vi "GetNodeList.vi"(8 "Status":T4[](array[typedef]), 10 "servers":T3[](array[typedef])) -> (1 "Topic Types":string[](array[string]), 3 "Published Topics":string[](array[string]))   [LabVIEW 2012]
doc: "Gets all topics that are published by this node."
uses:
  <userlib>/rosforlv/ROS/Code/Console/Servers/ServerSubs/MyState.ctl
  <userlib>/rosforlv/ROS/Code/Console/Servers/ServerSubs/ServoInfo.ctl
  <userlib>/rosforlv/ROS/Code/SubVIs/_ROSControl.ctl
  <userlib>/rosforlv/ROS/Code/SubVIs/_ROSDirection.ctl
panel:
  in  "ROS.Direction":T1
  in  "Node ROS":T2={"topic port"=0, "Node"="", "topic"="", "type"="", "node port"=0, "error "={"status"=FALSE, "code"=0, "source"=""}, "Direction"=enum."Node", "APIs"=[], "Update (ms)"=1, "write queue"=1}
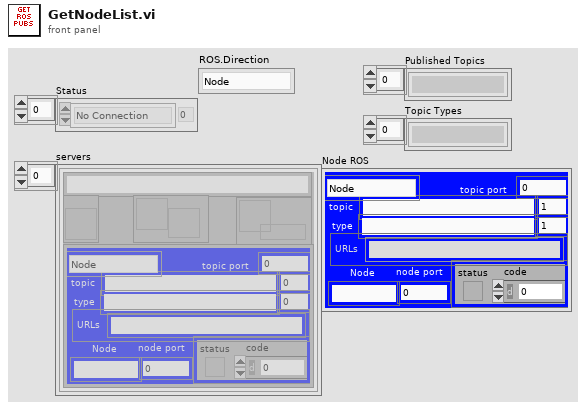
[diagram p1: front panel]
types:
  T1 = typedef "_ROSDirection.ctl" = enum16{"Node", "Publisher", "Subscriber", "Service Client"}
  T2 = typedef "_ROSControl.ctl" = cluster{"topic port":u16, "Node":string, "topic":string, "type":string, "node port":u32, "error ":errorcluster, "Direction":T1, "APIs":string[], "Update (ms)":u16, "write queue":u16}
  T3 = typedef "ServoInfo.ctl" = cluster{"vi name":string, "VI Refnum":refnum<vi>, "queue":refnum<queue>, "ROS":T2, "notifier":refnum<notifier>}
  T4 = typedef "MyState.ctl" = enum16{"No Connection", "Registered", "Connected", "Close"}
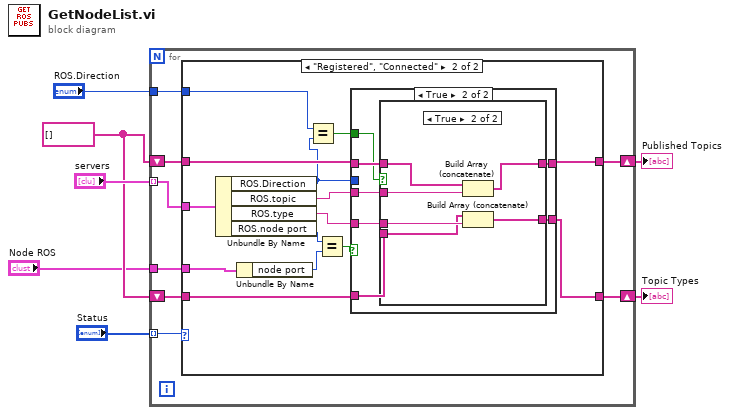
[diagram p0: block diagram]
diagram:
  w4 = string[] []
  n1 = for {
    tunnel: "servers" -> [w15] mode=indexing
    tunnel: "Status" -> [w9] mode=indexing
    shift-right: [w14] -> w5
    shift-left: w4 -> [w13]
    shift-right: [w12] -> w3
    shift-left: w4 -> [w11]
    tunnel: "Node ROS" -> [w10]
    tunnel: "ROS.Direction" -> [w8]
    n2 = case shown="\"Registered\", \"Connected\"" w9 {
      tunnel: w15 -> [_ w31]
      tunnel: [w17 w29] -> w14
      tunnel: w13 -> [w17 w28]
      tunnel: [w16 w26] -> w12
      tunnel: w11 -> [w16 w25]
      tunnel: w10 -> [_ w24]
      tunnel: w8 -> [_ w20]
      frame "No Connection", Default {
      }
      frame "Registered", "Connected" {
        n3 = Unbundle By Name(w31) -> ("ROS.Direction"=w19:T1, "ROS.topic"=w30:string, "ROS.type"=w27:string, "ROS.node port"=w22:u32)
        n4 = Unbundle By Name(w24) -> ("node port"=w21:u32)
        n5 = Equal?(x=w20, y=w19) -> (x = y?=w18:bool)
        n6 = Equal?(x=w22, y=w21) -> (x = y?=w23:bool)
        n7 = case shown="True" w23 {
          tunnel: w30 -> [_ w40]
          tunnel: [w33 w39] -> w29
          tunnel: w28 -> [w33 w38]
          tunnel: w19 -> [_ _]
          tunnel: w27 -> [_ w37]
          tunnel: [w32 w36] -> w26
          tunnel: w25 -> [w32 w35]
          tunnel: w18 -> [_ w34]
          frame False {
          }
          frame True {
            n8 = case shown="True" w34 {
              tunnel: w40 -> [_ w48]
              tunnel: [w42 w46] -> w39
              tunnel: w38 -> [w42 w47]
              tunnel: w37 -> [_ w45]
              tunnel: [w41 w44] -> w36
              tunnel: w35 -> [w41 w43]
              frame False {
              }
              frame True {
                n9 = Build Array (concatenate)(w47, w48) -> (w46:string[])
                n10 = Build Array (concatenate)(w43, w45) -> (w44:string[])
              }
            }
          }
        }
      }
    }
  }
  "Published Topics" <- w5
  "Topic Types" <- w3
